vi "UTIL_Get Screen Resolution v1_0_0.vi"(8 "error in (no error)":errorcluster) -> (0 "error out":errorcluster, 1 "height":i32, 2 "width":i32, 3 "screen size":i32)   [LabVIEW 2009]
doc: "UTIL_Get Screen Resolution v1_0_0.vi\n\nThis VI outputs an I32 that represents the screen size in use:\n\n0: smaller than 1024x768\n1: larger than 1024x768 but smaller than 1280x1024\n2: larger than 1280x1024\n\nAlso outputs two I32 that represent the exact Width and Height of the current monitor\n\nCreated 2006 by\n\nJ. Daren Suntych\nNational Analytics\n970-397-0764"
uses:
  user32.dll
panel:
  # "This VI outputs an I32 that represents the screen size in use:\n\n0:  smaller than 1024x768\n1:  larger than 1024x768 but smaller than 1280x1024\n2:  larger than 1280x1024"
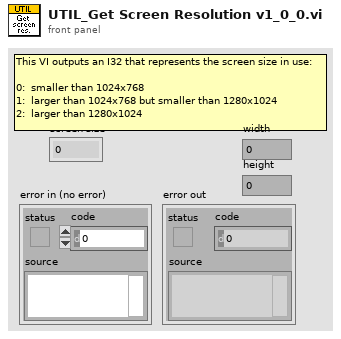
[diagram p1: front panel]
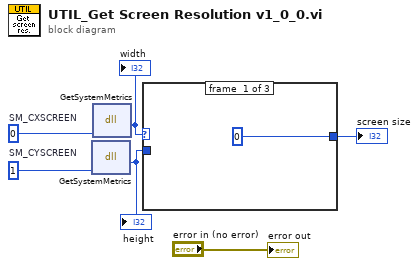
[diagram p0: block diagram]
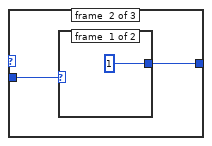
[diagram p2: hidden frame]
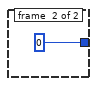
[diagram p3: hidden frame]
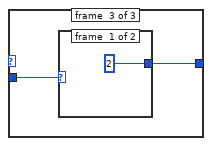
[diagram p4: hidden frame]
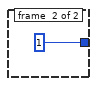
[diagram p5: hidden frame]
diagram:
  w3 = 1  # SM_CYSCREEN
  w4 = 0  # SM_CXSCREEN
  n1 = dll-call lib="user32.dll" fn="GetSystemMetrics"("parameter"=w3) -> ("screenHeight"=w1:i32)  [unwired: 4 in, 2 out]
  "height" <- w1
  n2 = dll-call lib="user32.dll" fn="GetSystemMetrics"("parameter"=w4) -> ("screenWidth"=w2:i32)  [unwired: 4 in, 2 out]
  "width" <- w2
  n3 = case shown="1280.." w2 {
    tunnel: [0 ("screen size") w9 w13] -> w6
    tunnel: w1 -> [_ w8 w12]
    frame #0 {
    }
    frame #1 {
      n4 = case shown="768.." w8 {
        tunnel: [1 ("screen size") 0 ("screen size")] -> w9
        frame #0 {
        }
        frame #1 {
        }
      }
    }
    frame #2 {
      n5 = case shown="1024.." w12 {
        tunnel: [2 ("screen size") 1 ("screen size")] -> w13
        frame #0 {
        }
        frame #1 {
        }
      }
    }
  }
  "screen size" <- w6
  "error out" <- "error in (no error)"
